vi "Match Suit.vi"(7 "SS Image Path":path=path "C:/PokerSS/ViewSonic SS2.png", 8 "error in":errorcluster, 10 "Suit Template":path=path "C:/Users/Bob Dabalina/Documents/Labview/Poker Hand2/Heart Template.png", 11 "ROI Descriptor":T1={"Global Rectangle"=[530, 711, 555, 739], "Contours"=[{"ID"=enum."External", "Type"=12, "Coordinates"=[530, 711, 555, 739, 0]}]} {"Contours"."Type" items=["No Selection", "Point", "Line", "Rectangle", "Oval", "Polygon", "Freehand Region", "Annulus", "Unused2", "Unused3", "Broken Line", "Freehand Line", "Rotated Rectangle"]}) -> (0 "error out":errorcluster, 2 "Suit Score":dbl, 3 "Suit Found?":bool)   [LabVIEW 2015]
uses:
  <vilib>/vision/NI_Vision_Development_Module.lvlib
panel:
  in  "Match Suit Threshold":sgl=900.0
  out "Image Out":T2(plugin-control)
  out "Matches":T3(array[cluster]) {"Bounding Box"."y" format="%.2f"; "Bounding Box"."x" format="%.2f"; "Position"."y" format="%.2f"; "Position"."x" format="%.2f"; "Score" format="%.2f"; "Scale" format="%.2f"; "Angle" format="%.2f"}
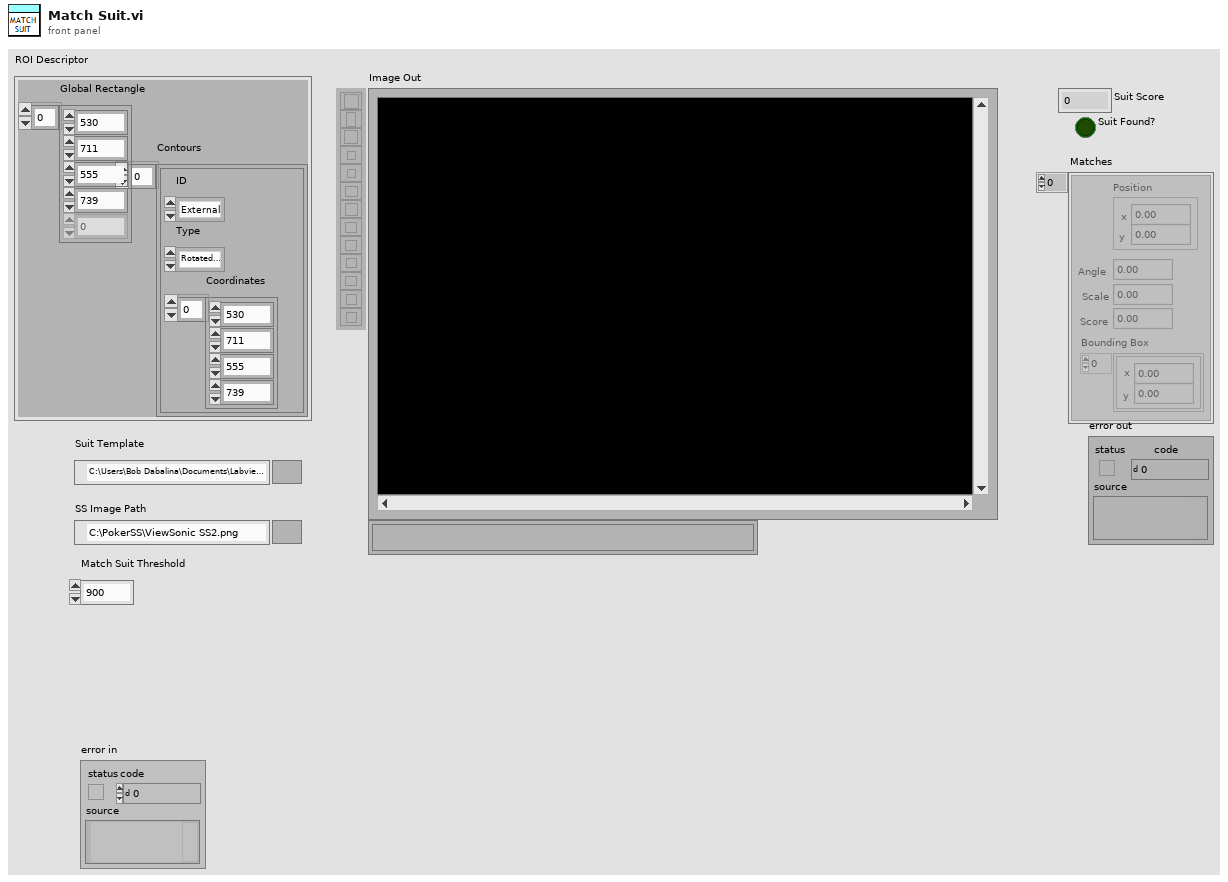
[diagram p1: front panel]
types:
  T1 = cluster{"Global Rectangle":i32[], "Contours":cluster{"ID":enum32{"External", "Internal"}, "Type":u32, "Coordinates":i32[]}[]}
  T2 = typedef "IMAQ Image.ctl" = refnum<image>
  T3 = cluster{"Position":cluster{"x":sgl, "y":sgl}, "Angle":sgl, "Scale":sgl, "Score":sgl, "Bounding Box":cluster{"x":sgl, "y":sgl}[]}[]
  T4 = cluster{"Number of Matches Requested":i32, "Minimum Match Score":sgl, "Angle Ranges":cluster{"Start Angle":sgl, "End Angle":sgl}[]}
  T5 = typedef "Image Type" = u32
  T6 = cluster{"Position":cluster{"x":sgl, "y":sgl}, "Angle":sgl, "Scale":sgl, "Score":sgl, "Bounding Box":cluster{"x":sgl, "y":sgl}[]}
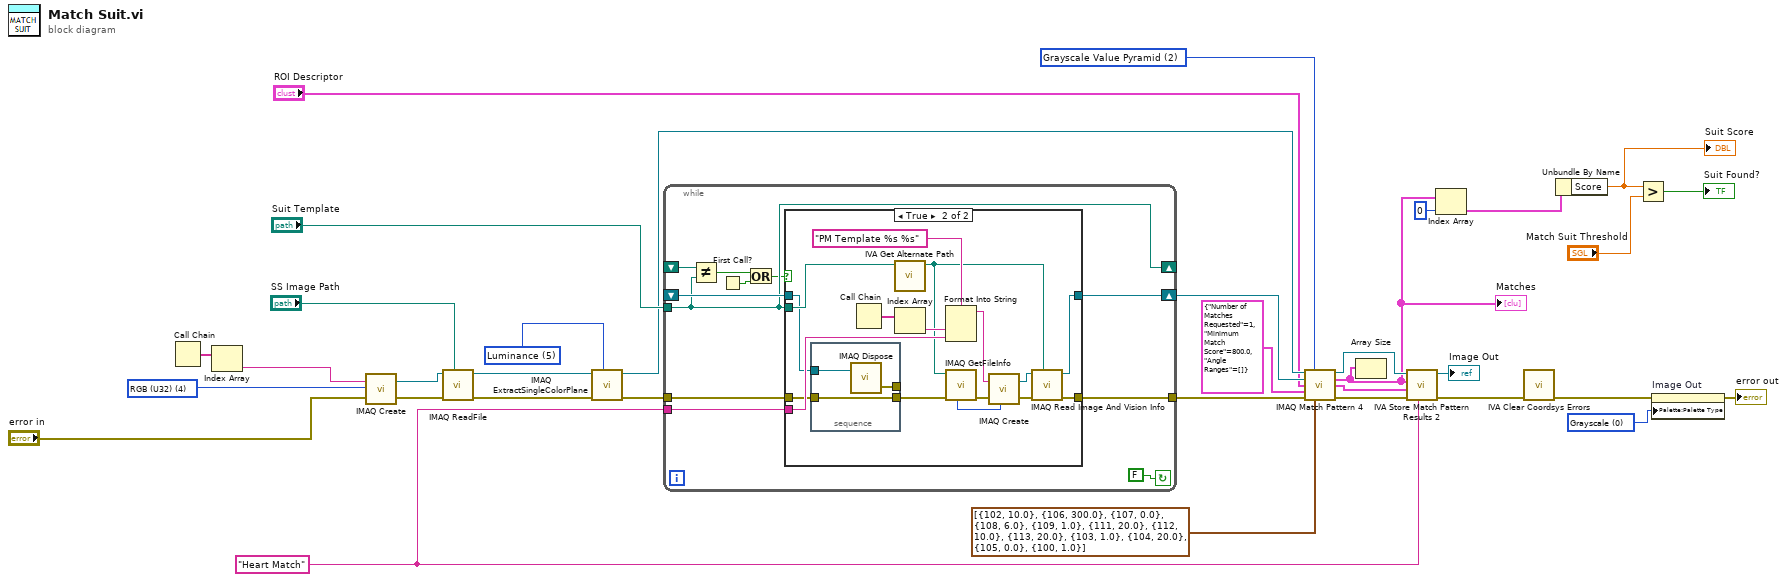
[diagram p0: block diagram]
diagram:
  w9 = u32 0 items=["Grayscale", "Binary", "Gradient", "Rainbow", "Temperature", "User Defined", "Binary 16 Bit", "Gradient 16 Bit", "Rainbow 16 Bit", "Temperature 16 Bit", "User Defined 16 Bit"] ("Palette Type")
  w20 = 2 items=["All", "Low Discrepancy Sampling", "Grayscale Value Pyramid", "Gradients Pyramid"] ("Algorithm")
  w18 = "Heart Match" ("Step Name")
  w27 = 5 items=["Red", "Green", "Blue", "Hue", "Saturation", "Luminance", "Value", "Intensity"] ("Color Plane")
  w28 = T5 4 items=["Grayscale (U8)", "Grayscale (I16)", "Grayscale (SGL)", "Complex (CSG)", "RGB (U32)", "HSL (U32)", "RGB (U64)", "Grayscale (U16)"] ("Image Type")
  n1 = Call Chain() -> (call chain=w30:string[])
  n2 = Index Array(array=w30) -> (element=w29:string)  [unwired: 1 in]
  n3 = call "IMAQ Create"("Image Name"=w29, "Image Type"=w28, "error in (no error)"="error in") -> ("New Image"=w33:T2, "error out"=w32:errorcluster)  [unwired: 1 in, 1 out]
  n4 = call "IMAQ ReadFile"("File Path"="SS Image Path", "error in (no error)"=w32, "Image"=w33) -> ("error out"=w34:errorcluster, "Image Out"=w26:T2)  [unwired: 2 in, 5 out]
  n5 = call "IMAQ ExtractSingleColorPlane"("Color Plane"=w27, "error in (no error)"=w34, "Image Src"=w26) -> ("error out"=w25:errorcluster, "Image Dst Out"=w23:T2)  [unwired: 1 in, 6 out]
  n6 = while {
    shift-right: [w45] -> w16
    shift-left: _ -> [w44]
    tunnel: [w42] -> w15
    tunnel: w25 -> [w41]
    tunnel: "Suit Template" -> [w38]
    tunnel: w18 -> [w40]
    shift-right: [w38] -> _
    shift-left: _ -> [w39]
    stop <- FALSE continue-if-true
    n7 = Not Equal?(x=w39, y=w38) -> (x != y?=w36:bool)
    n8 = First Call?() -> (First Call?: T/F=w37:bool)
    n9 = Or(x=w36, y=w37) -> (x .or. y?=w35:bool)
    n10 = case shown="True" w35 {
      tunnel: [w47 w61] -> w45
      tunnel: w44 -> [w47 w53]
      tunnel: [w46 w58] -> w42
      tunnel: w41 -> [w46 w52]
      tunnel: w38 -> [_ w54]
      tunnel: w40 -> [_ w55]
      frame False {
      }
      frame True {
        n11 = stacked-sequence {
          tunnel: w53 -> [w66]
          tunnel: w52 -> [w65]
          tunnel: [w65] -> w48
          tunnel: [w64] -> _
          frame #0 {
            n12 = call "IMAQ Dispose"("Image"=w66) -> ("error out"=w64:errorcluster)  [unwired: 2 in, 3 out]
          }
        }
        n13 = Call Chain() -> (call chain=w57:string[])
        n14 = call <vilib>:"IVA Get Alternate Path.vi"("Path In"=w54) -> ("Path Out"=w50:path)  [unwired: 10 out]
        n15 = Index Array(array=w57) -> (element=w56:string)  [unwired: 1 in]
        n16 = Format Into String(format string="PM Template %s %s" ("Image Name"), w56, w55) -> (resulting string=w63:string)  [unwired: 2 in, 1 out]
        n17 = call "IMAQ GetFileInfo"("error in (no error)"=w48, "File Path"=w50) -> ("error out"=w49:errorcluster, "Image Type"=w51:T5)  [unwired: 3 in, 5 out]
        n18 = call "IMAQ Create"("Image Name"=w63, "Image Type"=w51, "error in (no error)"=w49) -> ("New Image"=w60:T2, "error out"=w59:errorcluster)  [unwired: 1 in, 1 out]
        n19 = call "IMAQ Read Image And Vision Info"("File Path"=w50, "error in (no error)"=w59, "Image"=w60) -> ("error out"=w58:errorcluster, "Image Out"=w61:T2)  [unwired: 1 in, 6 out]
      }
    }
  }
  n20 = call "IMAQ Match Pattern 4"("Image"=w23, "Algorithm"=w20, "Template Image"=w16, "ROI Descriptor"="ROI Descriptor", "Parameters"=T4 {"Number of Matches Requested"=1, "Minimum Match Score"=800.0, "Angle Ranges"=[]}, "error in (no error)"=w15, "Advanced Options"=cluster{"Item":u16, "Value":dbl}[] [{"Item"=102, "Value"=10.0}, {"Item"=106, "Value"=300.0}, {"Item"=107, "Value"=0.0}, {"Item"=108, "Value"=6.0}, {"Item"=109, "Value"=1.0}, {"Item"=111, "Value"=20.0}, {"Item"=112, "Value"=10.0}, {"Item"=113, "Value"=20.0}, {"Item"=103, "Value"=1.0}, {"Item"=104, "Value"=20.0}, {"Item"=105, "Value"=0.0}, {"Item"=100, "Value"=1.0}]) -> ("Image (duplicate)"=w21:T2, "Matches (pixel)"=w6:T3, "Matches (real-world)"=w17:T3, "error out"=w22:errorcluster)  [unwired: 4 in, 1 out]
  "Matches" <- w6
  n21 = Array Size(array=w6) -> ()  [unwired: 1 out]
  n22 = call <vilib>:"IVA Store Match Pattern Results 2.vi"("Step Name"=w18, "error in (no error)"=w22, "Matches (real-world)"=w17, "Matches (pixel)"=w6, "Image in"=w21) -> ("error out"=w14:errorcluster, "Image dup"=→"Image Out":T2)  [unwired: 1 in, 4 out]
  n23 = Index Array(array=w6, index=0) -> (element=w5:T6)
  n24 = call <vilib>:"IVA Clear Coordsys Errors.vi"("error in (no error)"=w14) -> ("error out"=w13:errorcluster)  [unwired: 10 in]
  n25 = Unbundle By Name(w5) -> ("Score"=w1:sgl)
  "Suit Score" <- w1
  n26 = Greater?(x=w1, y="Match Suit Threshold") -> (0:→"Suit Found?":bool)
  n27 = property on="Image Out" class="ImageControl"(error in=w13, "Palette:Palette Type"=w9) -> (error out=→"error out":errorcluster)  [unwired: 1 in, 1 out]
